vi "Quadrature Decoder.vi"(9 "Reset":bool, 10 "B":bool, 11 "A":bool) -> (3 "Counter":i32)   [LabVIEW 2017]
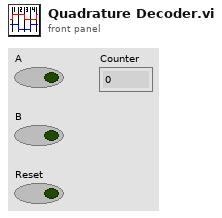
[diagram p1: front panel]
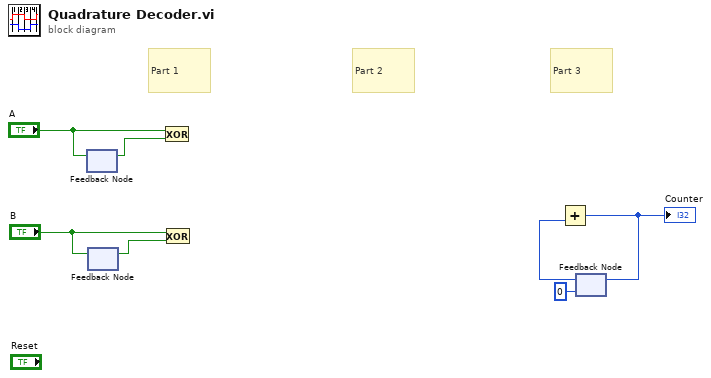
[diagram p0: block diagram]
diagram:
  # "Part 3"
  # "Part 2"
  # "Part 1"
  n1 = feedback #1() -> (w5:bool)  [unwired: 1 in]
  n2 = feedback-in #1("A") -> ()
  n3 = feedback #2() -> (w7:bool)  [unwired: 1 in]
  n4 = feedback-in #2("B") -> ()
  n5 = Exclusive Or(1:w5, 2:"A") -> ()  [unwired: 1 out]
  n6 = Exclusive Or(1:w7, 2:"B") -> ()  [unwired: 1 out]
  n7 = feedback #3(0) -> (w1:i32)
  n8 = Add(y=w1) -> (x+y=w3:i32)  [unwired: 1 in]
  "Counter" <- w3
  n9 = feedback-in #3(w3) -> ()
